vi "reverse black and white.vi"(11 "image data in":T1) -> (3 "image data out":T1)   [LabVIEW 2011]
uses:
  <vilib>/picture/picture.llb/imagedata.ctl
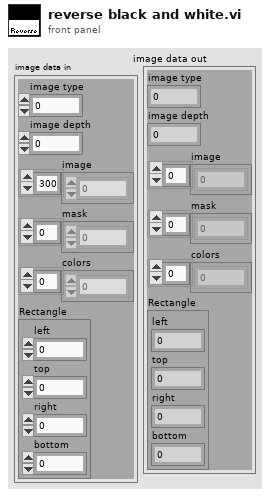
[diagram p1: front panel]
types:
  T1 = typedef "imagedata.ctl" = cluster{"image type":i32, "image depth":i32, "image":u8[], "mask":u8[], "colors":u32[], "Rectangle":cluster{"left":i16, "top":i16, "right":i16, "bottom":i16}}
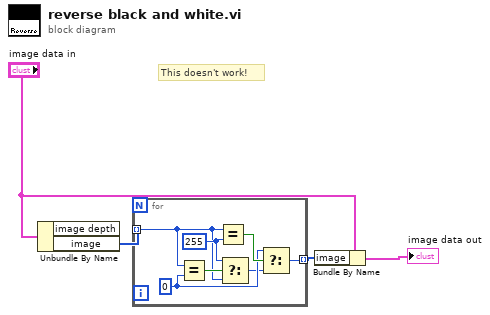
[diagram p0: block diagram]
diagram:
  # "This doesn't work!"
  n1 = Unbundle By Name("image data in") -> ("image"=w2:u8[])  [unwired: 1 out]
  n2 = for {
    tunnel: w2 -> [w7] mode=indexing
    tunnel: [w5] -> w3 mode=indexing
    w10 = u8 0 ("y")
    w8 = u8 255 ("y")
    n3 = Equal?(x=w7, y=w10) -> (x = y?=w9:bool)
    n4 = Equal?(x=w7, y=w8) -> (x = y?=w11:bool)
    n5 = Select(t=w8, s=w9, f=w7) -> (s? t:f=w6:u8)
    n6 = Select(t=w10, s=w11, f=w6) -> (s? t:f=w5:u8)
  }
  n7 = Bundle By Name(cluster="image data in", "image"=w3) -> (→"image data out":T1)
